vi "motor_get.vi"(6 "delay  (sec)":dbl=0.1 caption="Delay Time (s)", 8 "error in":errorcluster, 10 "command":string="IP", 11 "VISA in":refnum<visa-resource-name>) -> (0 "error out":errorcluster, 1 "return count":u32, 2 "return":string, 3 "VISA out":refnum<visa-resource-name>)   [LabVIEW 2019]
panel:
  out "bytes":u32
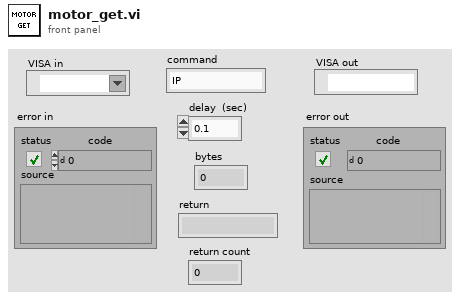
[diagram p1: front panel]
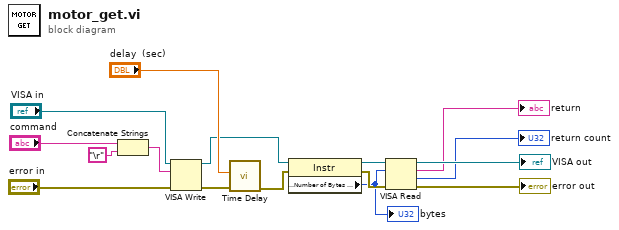
[diagram p0: block diagram]
diagram:
  n1 = Concatenate Strings("command", "\r") -> (w16:string)
  n2 = VISA Write(VISA resource name="VISA in", write buffer=w16, error in (no error)="error in") -> (VISA resource name out=w9:refnum<visa-resource-name>, error out=w12:errorcluster)  [unwired: 1 out]
  n3 = call "Time Delay"("error in (no error)"=w12, "Delay Time (s)"="delay  (sec)") -> ("error out"=w8:errorcluster)  [unwired: 9 in]
  n4 = property class="Instr"(reference=w9, error in=w8) -> (reference out=w7:refnum<visa-resource-name>, error out=w6:errorcluster, "Serial Settings:Number of Bytes at Serial Port"=w5:u32)
  "bytes" <- w5
  n5 = VISA Read(VISA resource name=w7, byte count=w5, error in (no error)=w6) -> (VISA resource name out=→"VISA out":refnum<visa-resource-name>, read buffer=→"return":string, return count=→"return count":u32, error out=→"error out":errorcluster)
